vi "Error Query.vi"(8 "error in (no error)":errorcluster, 11 "VISA resource name":refnum<visa-resource-name>) -> (0 "error out":errorcluster, 1 "Error Message":string, 2 "Error Code":i32[](array[numeric]), 3 "VISA resource name out":refnum<visa-resource-name>)   [LabVIEW 2014, in "Agilent U2000 Series.lvlib"]
doc: "Queries the instrument for any errors in the instrument's error queue. It will continue to read errors until all errors have been read from the instrument. Any errors will be returned in the <B>error out</B> control.\n\nNote:\nThis VI is called automatically by most driver VIs so it is not usually necessary to call this in an application."
uses:
  Agilent U2000 Series.lvlib
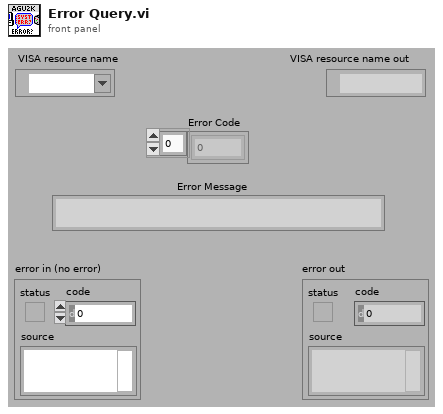
[diagram p1: front panel]
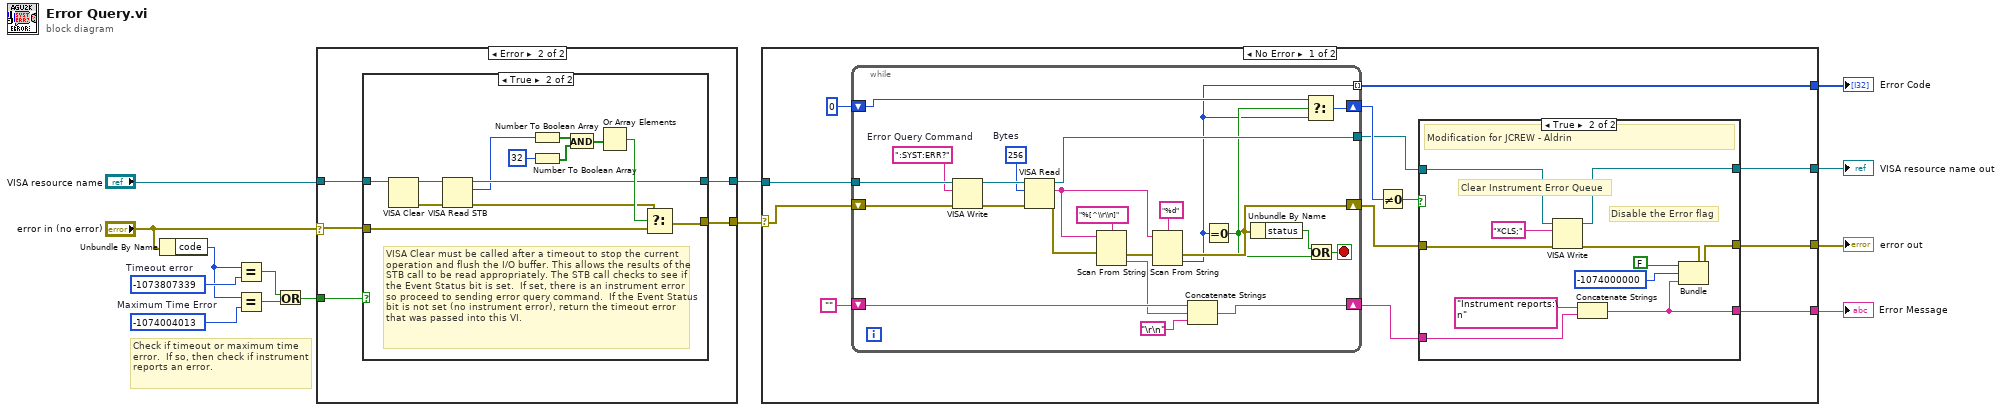
[diagram p0: block diagram]
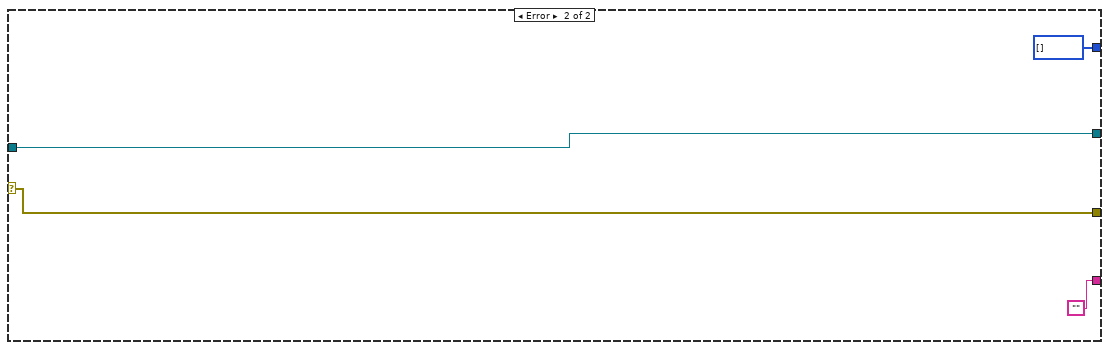
[diagram p5: hidden frame]
diagram:
  w5 = -1074004013  # Maximum Time Error
  w7 = -1073807339  # Timeout error
  # "Check if timeout or maximum time error.  If so, then check if instrument reports an error."
  n1 = Unbundle By Name("error in (no error)") -> ("code"=w6:i32)
  n2 = Equal?(x=w6, y=w7) -> (x = y?=w3:bool)
  n3 = Equal?(x=w6, y=w5) -> (x = y?=w4:bool)
  n4 = Or(x=w3, y=w4) -> (x .or. y?=w2:bool)
  n5 = case shown="Error" "error in (no error)" {
    selector: "error in (no error)" -> [w15 w19]
    tunnel: "VISA resource name" -> [w16 w21]
    tunnel: [w16 w20] -> w9
    tunnel: [w15 w18] -> w10
    tunnel: w2 -> [_ w17]
    frame No Error {
    }
    frame Error {
      n6 = case shown="True" w17 {
        tunnel: w21 -> [w23 w29]
        tunnel: [w23 w26] -> w20
        tunnel: w19 -> [w22 w32]
        tunnel: [w22 w31] -> w18
        frame False {
          # "Error code not a timeout, so best to pass on to user."
        }
        frame True {
          # "VISA Clear must be called after a timeout to stop the current operation and flush the I/O buffer. This allows the results of the  STB call to be read appropriately. The STB call checks to see if the Event Status bit is set.  If set, there is an instrument error so proceed to sending error query command.  If the Event Status bit is not set (no instrument error), return the timeout error that was passed into this VI."
          n7 = VISA Clear(VISA resource name=w29) -> (VISA resource name out=w28:refnum<visa-resource-name>, error out=w27:errorcluster)  [unwired: 1 in]
          n8 = VISA Read STB(8:w27, 11:w28) -> (0:w25:errorcluster, 2:w24:u16, 3:w26:refnum<visa-resource-name>)
          n9 = Number To Boolean Array(number=w24) -> (Boolean array=w33:bool[])
          n10 = Number To Boolean Array(number=32) -> (Boolean array=w35:bool[])
          n11 = And(x=w33, y=w35) -> (x .and. y?=w34:bool[])
          n12 = Or Array Elements(Boolean array=w34) -> (logical OR=w30:bool)
          n13 = Select(t=w25, s=w30, f=w32) -> (s? t:f=w31:errorcluster)
        }
      }
    }
  }
  n14 = case shown="No Error" w10 {
    selector: w10 -> [w44 w87]
    tunnel: [w41 w90] -> w14
    tunnel: w9 -> [w49 w90]
    tunnel: [w40 w87] -> w13
    tunnel: [w39 ""] -> w12
    tunnel: [w45 i32[] []] -> w11
    frame No Error {
      n15 = while {
        tunnel: [w86] -> w42
        tunnel: w49 -> [w85]
        shift-right: [w74] -> w38
        shift-left: "" -> [w77]
        shift-right: [w72] -> w46
        shift-left: 0 -> [w73]
        shift-right: [w70] -> w43
        shift-left: w44 -> [w71]
        tunnel: [w65] -> w45 mode=indexing
        stop <- w79 stop-if-true
        w83 = u32 256  # Bytes
        w81 = ":SYST:ERR?"  # Error Query Command
        n16 = VISA Write(VISA resource name=w85, write buffer=w81, error in (no error)=w71) -> (VISA resource name out=w84:refnum<visa-resource-name>, error out=w82:errorcluster)  [unwired: 1 out]
        n17 = VISA Read(VISA resource name=w84, byte count=w83, error in (no error)=w82) -> (VISA resource name out=w86:refnum<visa-resource-name>, read buffer=w64:string, error out=w69:errorcluster)  [unwired: 1 out]
        n18 = Scan From String(format string="%[^\\r\\n]", input string=w64, error in=w69) -> (error out=w68:errorcluster, output 1=w75:string)  [unwired: 1 in, 3 out]
        n19 = Scan From String(format string="%d", input string=w64, error in=w68) -> (error out=w70:errorcluster, output 1=w65:i32)  [unwired: 1 in, 3 out]
        n20 = Concatenate Strings(w77, w75, "\r\n") -> (w74:string)
        n21 = Equal To 0?(x=w65) -> (x = 0?=w66:bool)
        n22 = Unbundle By Name(w70) -> ("status"=w67:bool)
        n23 = Select(t=w73, s=w66, f=w65) -> (s? t:f=w72:i32)
        n24 = Or(x=w67, y=w66) -> (x .or. y?=w79:bool)
      }
      n25 = Not Equal To 0?(x=w46) -> (x != 0?=w37:bool)
      n26 = case shown="True" w37 {
        tunnel: w38 -> [w50 w62]
        tunnel: [w52 w56] -> w40
        tunnel: w43 -> [w52 w61]
        tunnel: w42 -> [w51 w59]
        tunnel: [w51 w58] -> w41
        tunnel: [w50 w53] -> w39
        frame False {
        }
        frame True {
          # "Disable the Error flag"
          # "Clear Instrument Error Queue"
          # "Modification for JCREW - Aldrin"
          n27 = VISA Write(VISA resource name=w59, write buffer="*CLS;", error in (no error)=w61) -> (VISA resource name out=w58:refnum<visa-resource-name>, error out=w57:errorcluster)  [unwired: 1 out]
          n28 = Concatenate Strings("Instrument reports:\n" ("Source"), w62) -> (w53:string)
          n29 = Bundle(cluster=w57, "status"=FALSE ("show call chain? (False)"), "code"=-1074000000 ("Code"), "source"=w53) -> (w56:errorcluster)
        }
      }
    }
    frame Error {
    }
  }
  "VISA resource name out" <- w14
  "error out" <- w13
  "Error Message" <- w12
  "Error Code" <- w11
